vi "Create-log-file.vi"(8 "error in (no error)":errorcluster, 11 "Errors in":T1) -> (0 "error out":errorcluster, 3 "Errors out":T1)   [LabVIEW 2013, in "Error-handling.lvlib" / "Errors.lvclass"]
uses:
  Errors.lvclass
  Object-reference.ctl
  Errors.lvclass/Errors.ctl
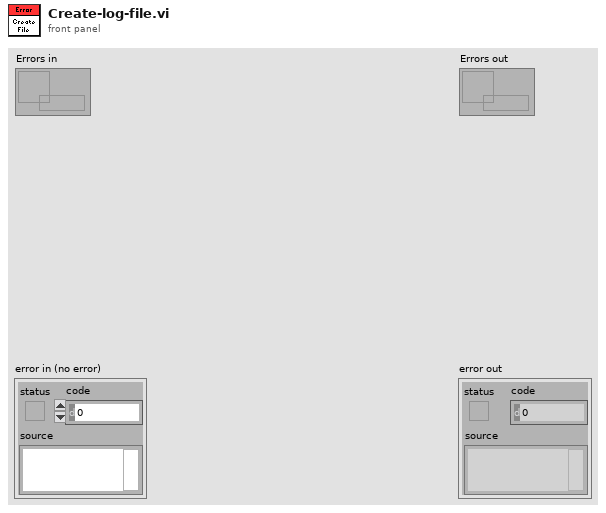
[diagram p1: front panel]
types:
  T1 = typedef "Error-handling.lvlib/Errors.lvclass/Object-reference.ctl" = refnum<data-value>
  T2 = enum16{"open", "replace", "create", "open or create", "replace or create", "replace or create with confirmation"}
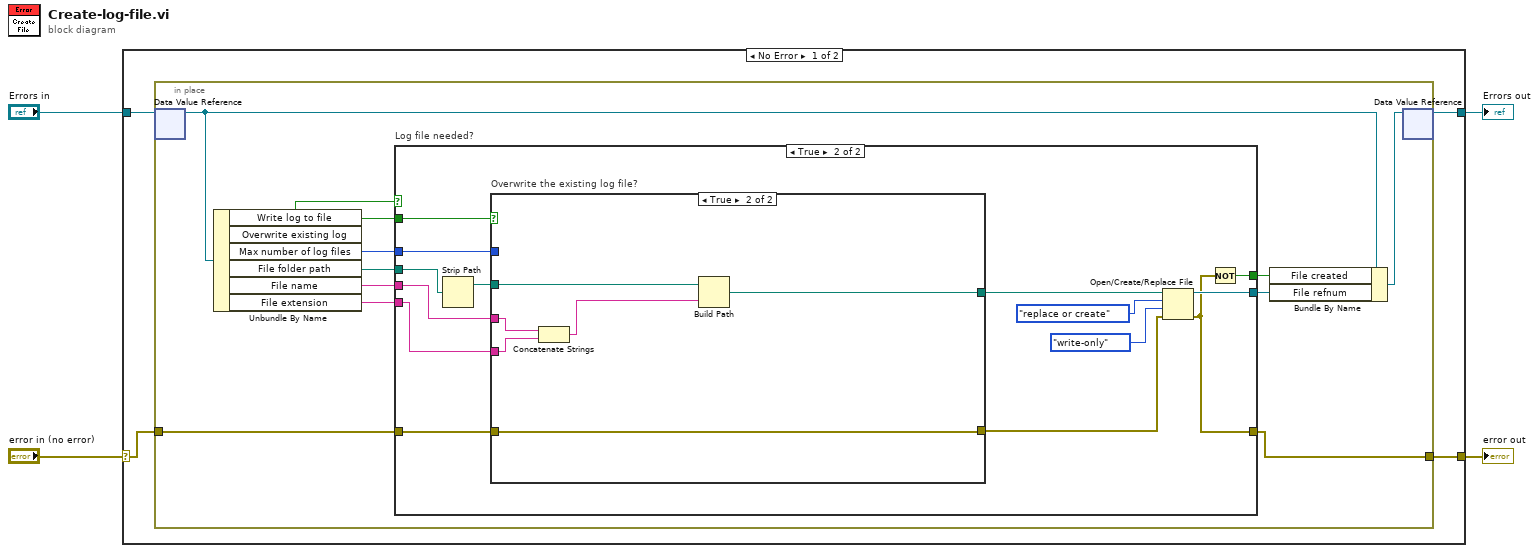
[diagram p0: block diagram]
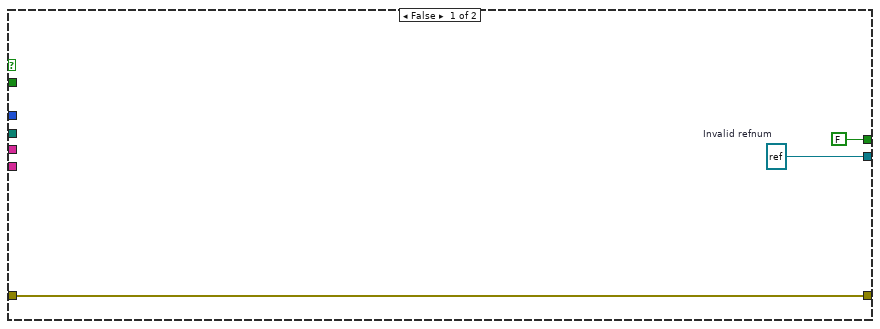
[diagram p2: hidden frame]
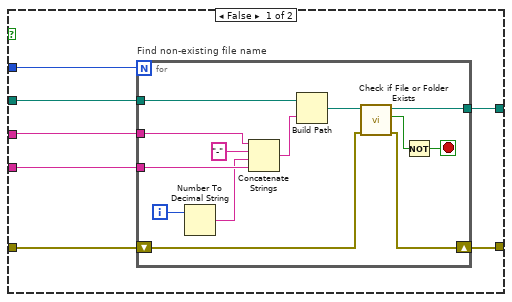
[diagram p3: hidden frame]
diagram:
  n1 = case shown="No Error" "error in (no error)" {
    selector: "error in (no error)" -> [w8 w65]
    tunnel: [w7 w65] -> w3
    tunnel: [w5 w64] -> w1
    tunnel: "Errors in" -> [w6 w64]
    frame No Error {
      n2 = in-place {
        in-place-border: w8 -> [w13]
        in-place-border: [w12] -> w7
        n3 = in-place-dvr #1(w6) -> (w10:refnum<class "Errors.lvclass">)  [unwired: 1 out]
        n4 = Unbundle By Name(w10) -> ("Write log to file"=w20:bool, "Overwrite existing log"=w18:bool, "Max number of log files"=w11:i32, "File folder path"=w19:path, "File name"=w17:string, "File extension"=w16:string)
        n5 = case "Log file needed?" shown="True" w20 {
          tunnel: w19 -> [_ w37]
          tunnel: w18 -> [_ w36]
          tunnel: w13 -> [w23 w34]
          tunnel: [w23 w27] -> w12
          tunnel: [w22 w29] -> w14
          tunnel: [FALSE w28] -> w15
          tunnel: w17 -> [_ w26]
          tunnel: w16 -> [_ w25]
          tunnel: w11 -> [_ w24]
          frame False {
            w22 = refnum<file> refnum  # Invalid refnum
          }
          frame True {
            n6 = Strip Path(path=w37) -> (stripped path=w35:path)  [unwired: 1 out]
            n7 = case "Overwrite the existing log file?" shown="True" w36 {
              tunnel: [w41 w62] -> w31
              tunnel: w35 -> [w44 w63]
              tunnel: w34 -> [w43 w61]
              tunnel: [w42 w61] -> w30
              tunnel: w26 -> [w40 w60]
              tunnel: w25 -> [w39 w59]
              tunnel: w24 -> [w38 _]
              frame False {
                n8 = for "Find non-existing file name" {
                  N: w38 -> [_]
                  tunnel: w44 -> [w57]
                  tunnel: w39 -> [w53]
                  tunnel: w40 -> [w54]
                  tunnel: [w51] -> w41
                  shift-right: [w47] -> w42
                  shift-left: w43 -> [w48]
                  i -> [w56]
                  stop <- w49 stop-if-true
                  n9 = Number To Decimal String(number=w56) -> (decimal integer string=w46:string)  [unwired: 1 in]
                  n10 = Concatenate Strings(w54, "-" ("string"), w46, w53) -> (w55:string)
                  n11 = Build Path(base path=w57, name or relative path=w55) -> (appended path=w52:path)
                  n12 = call <vilib>:"Check if File or Folder Exists.vi"("error in (no error)"=w48, "path"=w52) -> ("error out"=w47:errorcluster, "file or folder exists?"=w50:bool, "dup path"=w51:path)  [unwired: 7 in]
                  n13 = Not(x=w50) -> (.not. x?=w49:bool)
                }
              }
              frame True {
                n14 = Concatenate Strings(w60, w59) -> (w58:string)
                n15 = Build Path(base path=w63, name or relative path=w58) -> (appended path=w62:path)
              }
            }
            n16 = Open/Create/Replace File(file path (use dialog)=w31, error in=w30, operation (0:open)=T2."replace or create", access (0:read/write)=enum16{"read/write", "read-only", "write-only"}."write-only") -> (refnum out=w29:refnum<file>, error out=w27:errorcluster)  [unwired: 2 in, 1 out]
            n17 = Not(x=w27) -> (.not. x?=w28:bool)
          }
        }
        n18 = Bundle By Name(cluster=w10, "File created"=w15, "File refnum"=w14) -> (w9:refnum<class "Errors.lvclass">)
        n19 = in-place-dvr #1(w9) -> (w5:T1)  [unwired: 1 out]
      }
    }
    frame Error {
    }
  }
  "error out" <- w3
  "Errors out" <- w1
